vi "RandNRunningAvg.vi"() -> ()   [LabVIEW 2019]
panel:
  out "Random Plot":cluster{"number: 0 to 1":dbl, dbl}(graph)={"number: 0 to 1"=0.9309795521473752, 0.49464521849658566}
  in  "stop":bool
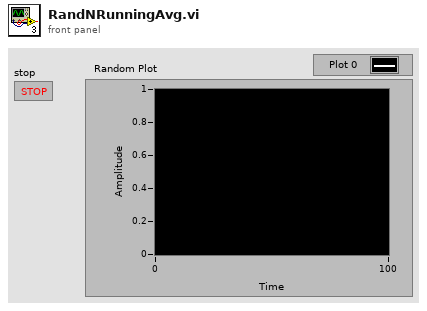
[diagram p1: front panel]
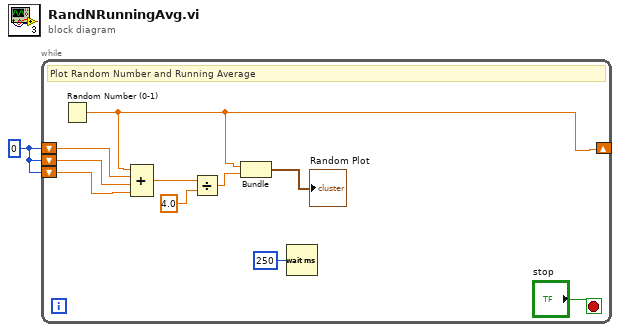
[diagram p0: block diagram]
diagram:
  w1 = 0
  n1 = while "Plot Random Number and Running Average" {
    shift-right: [w2] -> _
    shift-left: w1 -> [w10]
    shift-left: w1 -> [w9]
    shift-left: w1 -> [w8]
    stop <- "stop" stop-if-true
    # "Plot Random Number and Running Average"
    n2 = Random Number (0-1)() -> (number: 0 to 1=w2:dbl)
    n3 = Compound Arithmetic op=ADD(w2, w8, w9, w10) -> (w7:dbl)
    n4 = Divide(x=w7, y=4.0) -> (x/y=w5:dbl)
    n5 = Bundle("number: 0 to 1"=w2, w5) -> (→"Random Plot":cluster{"number: 0 to 1":dbl, dbl})  [unwired: 1 in]
    n6 = Wait (ms)(milliseconds to wait=u32 250) -> ()  [unwired: 1 out]
  }
